vi "Shooter (Gathering).vi"(1 "Execute":bool=TRUE) -> (4 "Done Executing":bool)   [LabVIEW 2011]
uses:
  Globals/Jaguar Commands.vi
  Globals/Shooter Gathering Velocity.vi
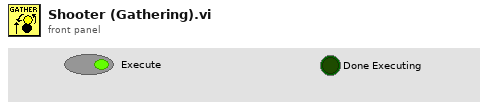
[diagram p1: front panel]
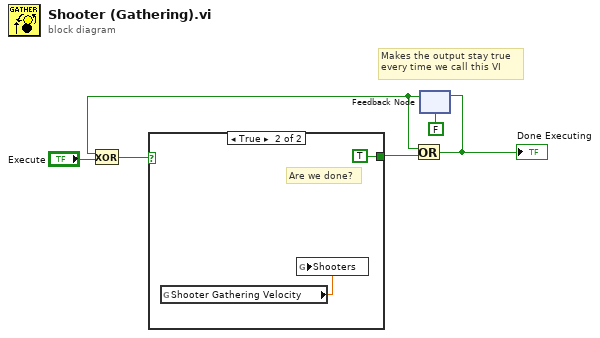
[diagram p0: block diagram]
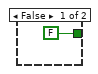
[diagram p2: hidden frame]
diagram:
  # "Makes the output stay true\nevery time we call this VI"
  n1 = feedback #1(FALSE) -> (w2:bool)
  n2 = Exclusive Or(1:"Execute", 2:w2) -> (0:w6:bool)
  n3 = case shown="True" w6 {
    tunnel: [FALSE TRUE] -> w4
    frame False {
    }
    frame True {
      # "Are we done?"
      n4 = global read "Shooter Gathering Velocity.vi" "Shooter Gathering Velocity"() -> (w8:dbl)
      n5 = global write "Jaguar Commands.vi" "Shooters"(w8) -> ()
    }
  }
  n6 = Or(x=w2, y=w4) -> (x .or. y?=w1:bool)
  "Done Executing" <- w1
  n7 = feedback-in #1(w1) -> ()
